vi "Set Position Setpoint.vi"(8 "error in (no error)":errorcluster, 10 "position (m)":dbl, 11 "KUKA youBot gripper motor_EtherCAT in":refnum<class "NI_Robotics_KUKA youBot Gripper Motor_EtherCAT.lvclass">) -> (0 "error out":errorcluster, 3 "KUKA youBot gripper motor_EtherCAT out":refnum<class "NI_Robotics_KUKA youBot Gripper Motor_EtherCAT.lvclass">)   [LabVIEW 2017, in "NI_Robotics_KUKA youBot Host.lvlib" / "NI_Robotics_KUKA youBot Gripper Motor_EtherCAT.lvclass"]
uses:
  <vilib>/robotics/KUKA youBot/Motor/Gripper Motor EtherCAT/NI_Robotics_KUKA youBot Gripper Motor_EtherCAT.lvclass
  c:/Program Files (x86)/National Instruments/LabVIEW 2017/vi.lib/robotics/KUKA youBot/Motor/Gripper Motor/NI_Robotics_KUKA youBot Gripper Motor.lvclass
  <vilib>/robotics/KUKA youBot/Motor/Gripper Motor EtherCAT/NI_Robotics_KUKA youBot Gripper Motor_EtherCAT.lvclass/NI_Robotics_KUKA youBot Gripper Motor_EtherCAT.ctl
  <vilib>/robotics/KUKA youBot/EtherCAT/EtherCAT Command.ctl
  <vilib>/robotics/KUKA youBot/EtherCAT/CmdCtrls/Param Cmd.ctl
  <vilib>/robotics/KUKA youBot/Motor/Gripper Motor/NI_Robotics_KUKA youBot Gripper Motor.lvclass
  <vilib>/robotics/KUKA youBot/NI_Robotics_KUKA youBot Host.lvlib
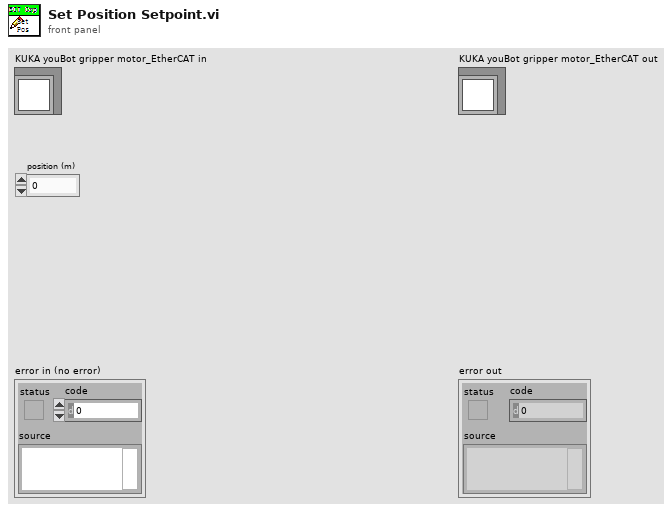
[diagram p1: front panel]
types:
  T1 = typedef "NI_Robotics_KUKA youBot Host.lvlib/EtherCAT Command.ctl" = cluster{"Module":u8, "Cmd":T2, "Type":u8, "Bank":u8, "Val":u32}
  T2 = typedef "NI_Robotics_KUKA youBot Host.lvlib/Param Cmd.ctl" = u8
  T3 = typedef "NI_Robotics_KUKA youBot Host.lvlib/Mater Handler.ctl" = i32
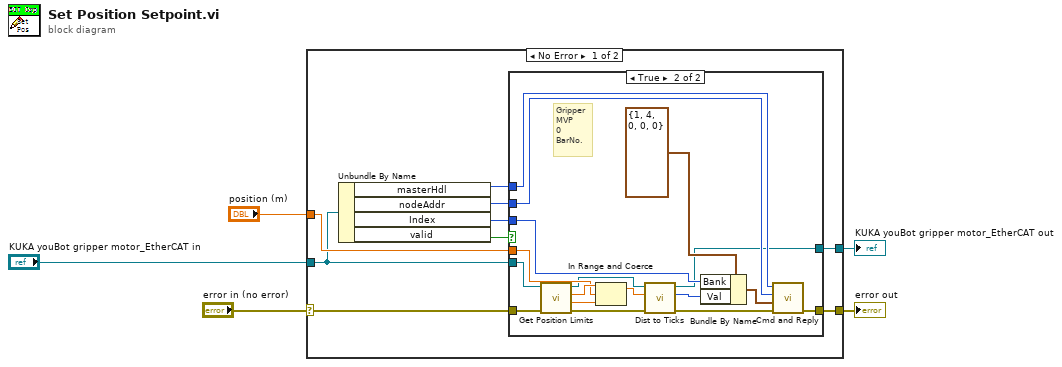
[diagram p0: block diagram]
diagram:
  n1 = case shown="No Error" "error in (no error)" {
    selector: "error in (no error)" -> [w14 w34]
    tunnel: "KUKA youBot gripper motor_EtherCAT in" -> [w12 w35]
    tunnel: "position (m)" -> [w13 _]
    tunnel: [w8 w35] -> w2
    tunnel: [w7 w34] -> w1
    frame No Error {
      n2 = Unbundle By Name(w12) -> ("masterHdl"=w11:T3, "nodeAddr"=w10:u16, "Index"=w9:i32, "valid"=w6:bool)
      n3 = case shown="True" w6 {
        tunnel: w14 -> [w15 w33]
        tunnel: w13 -> [_ w30]
        tunnel: w12 -> [w16 w25]
        tunnel: w11 -> [_ w24]
        tunnel: w10 -> [_ w23]
        tunnel: w9 -> [_ w21]
        tunnel: [w16 w18] -> w8
        tunnel: [w15 w17] -> w7
        frame False {
        }
        frame True {
          # "Gripper\nMVP\n0\nBarNo."
          n4 = call <vilib>:"Get Position Limits.vi"("error in (no error)"=w33, "KUKA youBot gripper motor in"=w25) -> ("error out"=w27:errorcluster, "min dist (m)"=w31:dbl, "max dist (m)"=w32:dbl, "KUKA youBot gripper motor out"=w29:refnum<class "NI_Robotics_KUKA youBot Gripper Motor_EtherCAT.lvclass">)  [unwired: 6 in]
          n5 = In Range and Coerce(upper limit=w32, x=w30, lower limit=w31) -> (coerced(x)=w28:dbl)  [unwired: 1 out]
          n6 = call <vilib>:"Dist to Ticks.vi"("error in (no error)"=w27, "distance (m)"=w28, "KUKA youBot gripper motor_EtherCAT in"=w29) -> ("error out"=w26:errorcluster, "ticks"=w20:i32, "KUKA youBot gripper motor_EtherCAT out"=w18:refnum<class "NI_Robotics_KUKA youBot Gripper Motor_EtherCAT.lvclass">)  [unwired: 6 in]
          n7 = Bundle By Name(cluster=T1 {"Module"=1, "Cmd"=4, "Type"=0, "Bank"=0, "Val"=0} ("EtherCAT Command"), "Bank"=w21, "Val"=w20) -> (w19:T1)
          n8 = call <vilib>:"Cmd and Reply.vi"("error in (no error)"=w26, "EtherCAT command"=w19, "nodeAddr in"=w23, "masterHdl in"=w24) -> ("error out"=w17:errorcluster)  [unwired: 3 in, 4 out]
        }
      }
    }
    frame Error {
    }
  }
  "error out" <- w1
  "KUKA youBot gripper motor_EtherCAT out" <- w2
